vi "GDF File Reader.vi"() -> ()   [LabVIEW 2016]
uses:
  GDFv1.x File Reader/_vlib/GDFv1.x.lvclass
  GDFv1.x File Reader/_vlib/GDFv1.x.lvclass/GDFv1.x.ctl
  GDF File Reader.lvlib
panel:
  out "Application state info":string caption="Состояние обработки"
  in  "Stop Button":bool
  in  "Tab Control":enum32{"График ЭЭГ", "Таблица событий"}(tab)
  in  "Previous Dataset":bool
  in  "Next Dataset":bool
  out "EEG Graph":waveform(dbl)[](graph) caption="График ЭЭГ"
  out "Selected path":path caption="Путь к файлу"
  out "Sample Rate":dbl caption="Частота" format="%#_3f"
  out "Number of channels":i64 caption="Число каналов"
  out "Patient identificator":string="                                      " caption="Испытуемый"
  in  "Number of Trials in File":i32 caption="Число проб в XML файле"
  in  "Event Duration (in seconds)":dbl=1.0 caption="Продолжительность, с"
  out "Number of Events":i32 caption="Число проб выбранного типа"
  in  "Select Event Type":string(combo) caption="Выберите тип событий"
  in  "Save Events":bool caption="Сохранить пробы в XML"
  in  "Multicolumn Listbox":i32[](listbox) caption="Таблица событий"
  # "This VI is a part of BCI Design library, http://www.ru-bci.org \nCopyright © 2020, Sotnikov Peter, All rights reserved. License: GNU GPLv3"
  # "Hz"
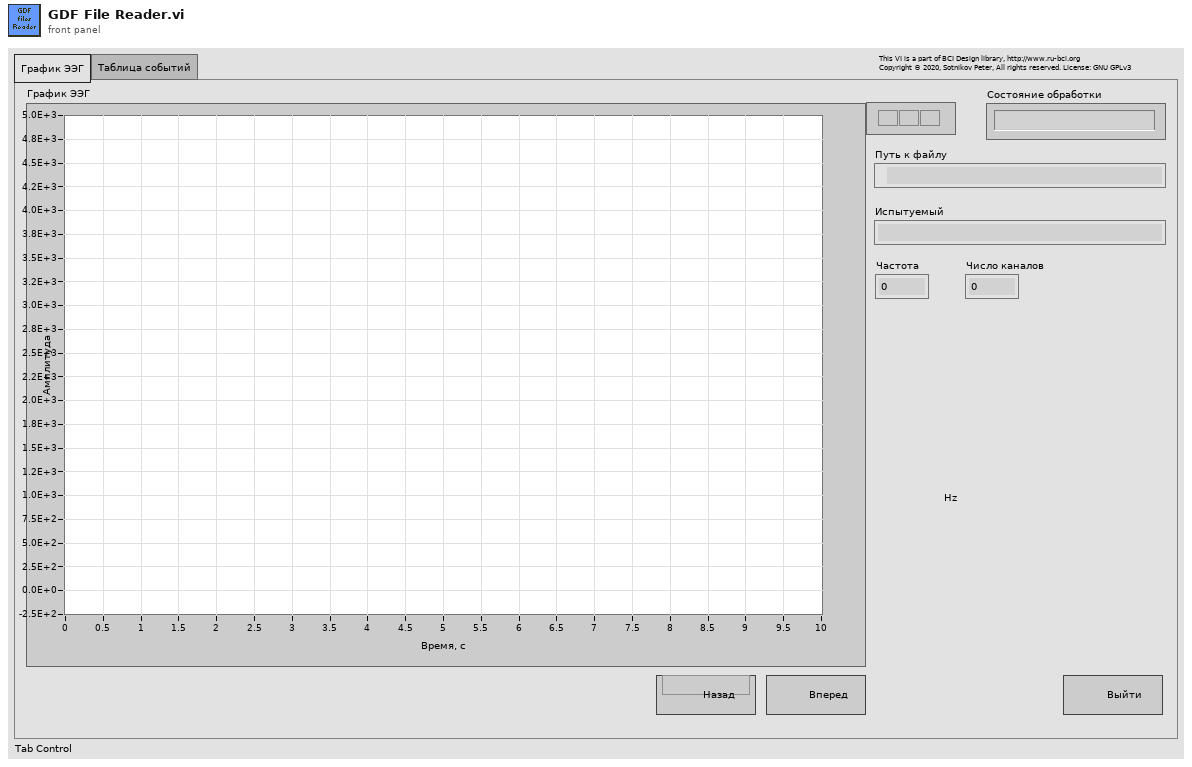
[diagram p1: front panel]
types:
  T1 = typedef "GDF File Reader.lvlib/GdfHeader1.ctl" = cluster{"Version identificator":string, "Patient identificator":string, "Recording identificator":string, "StartDateTime":timestamp, "Header record length":i64, "Equipment Provider":u64, "Laboratory":u64, "Technician":u64, "Number of data records":i64, "Duration of a data record":cluster{"Numerator":u32, "Denominator":u32}, "Number of signals":u32}
  T2 = typedef "GDF File Reader.lvlib/GdfHeader2.ctl" = cluster{"Channel labels":string[], "Transduser types":string[], "Physical dimensions":string[], "Physical lows":dbl[], "Physical highs":dbl[], "Digital lows":dbl[], "Digital highs":dbl[], "Channels Pre-filtering":string[], "Number of samples":u32[], "Channel types":u32[], "Addons":string[]}
  T3 = typedef "GDF File Reader.lvlib/EventDataType.ctl" = cluster{"Position (in samples)":u32, "EventType":string, "Channel":u16, "Duration (in samples)":u32}
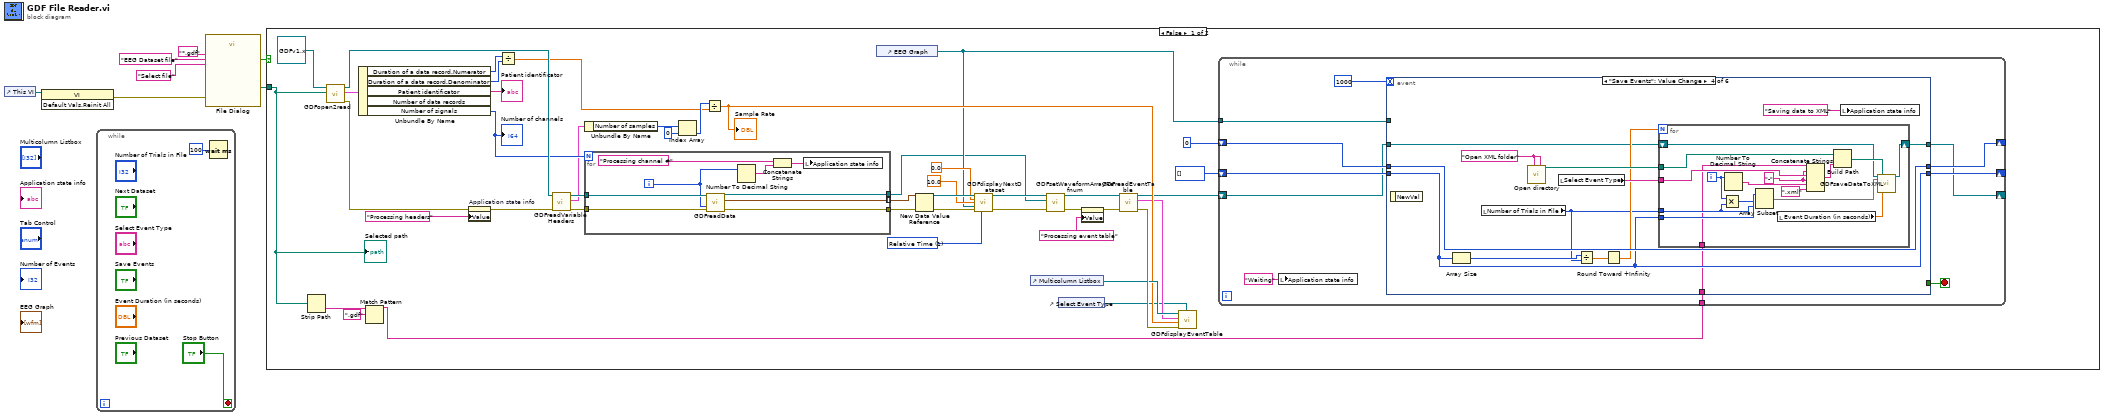
[diagram p0: block diagram]
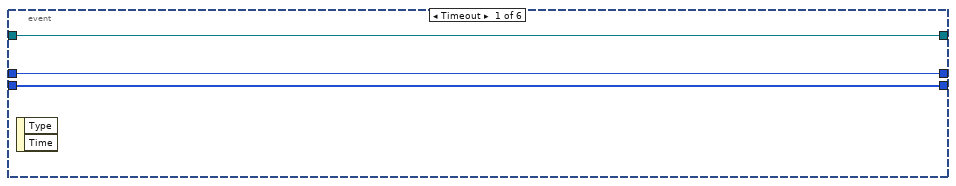
[diagram p2: hidden frame]
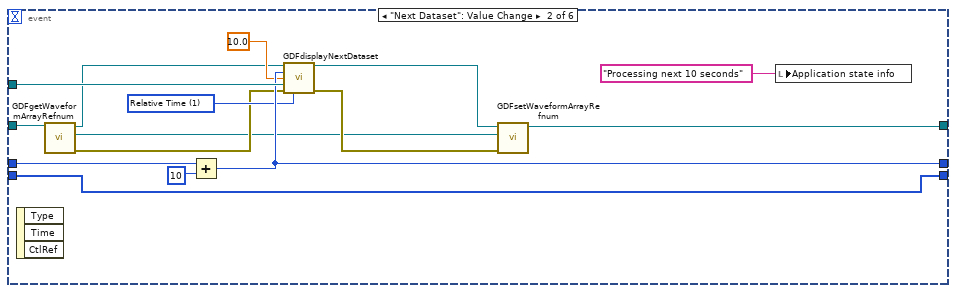
[diagram p3: hidden frame]
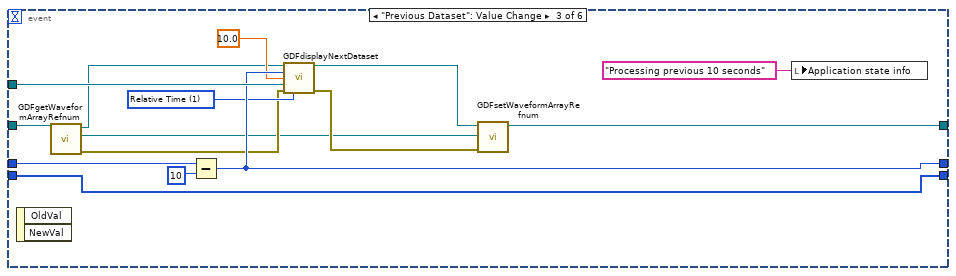
[diagram p4: hidden frame]
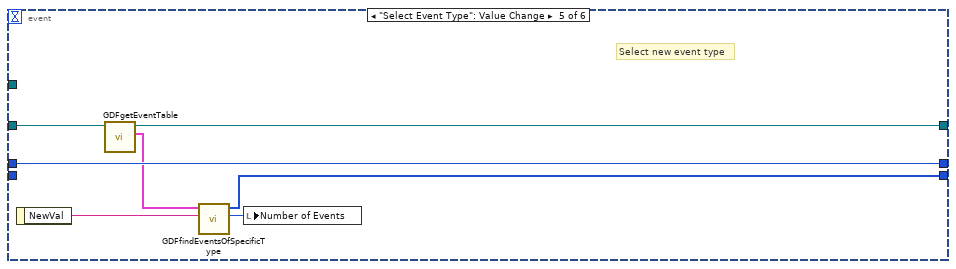
[diagram p5: hidden frame]
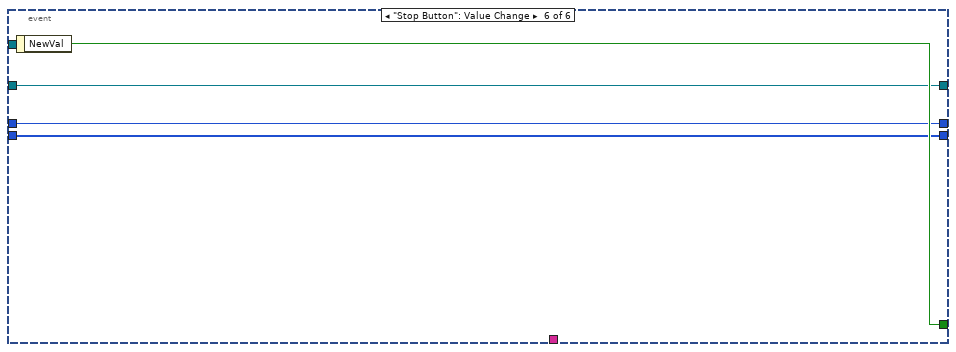
[diagram p6: hidden frame]
diagram:
  n1 = control-ref of="This VI"() -> (w2:refnum<vi>)
  n2 = invoke class="VI" method="Default Vals.Reinit All"(reference=w2) -> (error out=w1:errorcluster)  [unwired: 2 in, 2 out]
  n3 = while {
    stop <- "Stop Button" stop-if-true
    n4 = Wait (ms)(milliseconds to wait=u32 100) -> ()  [unwired: 1 out]
  }
  n5 = call "File Dialog"("button label"="Select file", "error in"=w1, "pattern (all files)"="*.gdf", "pattern label"="EEG Dataset file") -> ("selected path"=w4:path, "cancelled"=w5:bool)  [unwired: 8 in, 2 out]
  n6 = case shown="False" w5 {
    tunnel: w4 -> [w13 _]
    frame False {
      w24 = u16 1 items=["Samples", "Relative Time"] ("start/duration format")
      n7 = Strip Path(path=w13) -> (name=w12:string)  [unwired: 1 out]
      n8 = call "GDFopen2read.vi"("File path in"=w13, "GDFv1.x.lvclass in"=refnum<class "GDFv1.x.lvclass"> refnum ("GDFv1.x.lvclass")) -> ("error out"=w50:errorcluster, "GDF_header1"=w32:T1, "GDFv1.x.lvclass out"=w53:refnum<class "GDFv1.x.lvclass">)  [unwired: 7 in]
      n9 = Unbundle By Name(w32) -> ("Duration of a data record.Numerator"=w45:u32, "Duration of a data record.Denominator"=w44:u32, "Patient identificator"=→"Patient identificator":string, "Number of signals"=w36:u32)  [unwired: 1 out]
      "Number of channels" <- w36
      n10 = Match Pattern(string=w12, regular expression=".gdf") -> (before substring=w10:string)  [unwired: 1 in, 3 out]
      n11 = property on="Application state info" class="Str"(error in=w50, "Value"="Processing headers" ("Application state info")) -> (error out=w49:errorcluster)  [unwired: 1 in, 1 out]
      n12 = Divide(x=w45, y=w44) -> (x/y=w42:dbl)
      n13 = call "GDFreadVariableHeaders.vi"("error in"=w49, "GDFv1.x.lvclass in"=w53) -> ("error out"=w52:errorcluster, "GDFHeader2 out"=w31:T2, "GDFv1.x.lvclass out"=w51:refnum<class "GDFv1.x.lvclass">)  [unwired: 7 in]
      n14 = Unbundle By Name(w31) -> ("Number of samples"=w47:u32[])
      n15 = for {
        N: w36 -> [_]
        tunnel: w52 -> [w146]
        tunnel: w51 -> [w145]
        tunnel: [w144] -> w17
        tunnel: [w139] -> w30
        tunnel: [w138] -> w29 mode=indexing
        i -> [w141]
        n16 = call "GDFreadData.vi"("GDFv1.x.lvclass in"=w145, "Channel Number"=w141, "error in"=w146) -> ("GDFv1.x.lvclass out"=w144:refnum<class "GDFv1.x.lvclass">, "waveform out"=w138:waveform(dbl), "error out"=w139:errorcluster)  [unwired: 10 in]
        n17 = Number To Decimal String(number=w141) -> (decimal integer string=w140:string)  [unwired: 1 in]
        n18 = Concatenate Strings("Processing channel #" ("string"), w140) -> (w143:string)
        n19 = local write "Application state info"(w143) -> ()
      }
      n20 = Index Array(array=w47, index=0) -> (element=w43:u32)
      n21 = Divide(x=w43, y=w42) -> (x/y=w37:dbl)
      "Sample Rate" <- w37
      n22 = control-ref of="EEG Graph"() -> (w23:refnum<vi>)
      n23 = New Data Value Reference(data value=w29, error in=w30) -> (data value reference=w27:refnum<data-value>, error out=w28:errorcluster)
      n24 = call "GDFdisplayNextDataset.vi"("data value reference in"=w27, "Start"=0.0, "Duration"=10.0, "Waveform Graph Refnum in"=w23, "error in (no error)"=w28, "start/duration format"=w24) -> ("data value reference out"=w18:refnum<data-value>, "error out"=w20:errorcluster)  [unwired: 8 in]
      n25 = control-ref of="Multicolumn Listbox"() -> (w38:refnum<vi>)
      n26 = call "GDFsetWaveformArrayRefnum.vi"("error in (no error)"=w20, "GDFv1.x in"=w17, "Waveform Array Refnum in"=w18) -> ("error out"=w19:errorcluster, "GDFv1.x out"=w16:refnum<class "GDFv1.x.lvclass">)  [unwired: 7 in]
      n27 = control-ref of="Select Event Type"() -> (w22:refnum<vi>)
      n28 = property on="Application state info" class="Str"(error in=w19, "Value"="Processing event table") -> (error out=w34:errorcluster)  [unwired: 1 in, 1 out]
      n29 = call "GDFreadEventTable.vi"("error in"=w34, "GDFv1.x.lvclass in"=w16) -> ("error out"=w39:errorcluster, "Array of Events"=w33:T3[], "GDFv1.x.lvclass out"=w15:refnum<class "GDFv1.x.lvclass">)  [unwired: 6 in, 1 out]
      n30 = call "GDFdisplayEventTable.vi"("Select Event Type"=w22, "error in (no error)"=w39, "Samplerate"=w37, "Array of Events in"=w33, "Multicolumn Listbox in"=w38) -> ()  [unwired: 6 in, 1 out]
      n31 = while {
        shift-right: [w62] -> _
        shift-left: 0 -> [w61]
        tunnel: w23 -> [w59]
        shift-right: [w57] -> _
        shift-left: i32[] [] -> [w58]
        shift-right: [w55] -> _
        shift-left: w15 -> [w56]
        tunnel: w10 -> [w54]
        stop <- w63 stop-if-true
        n32 = local write "Application state info"("Waiting" ("Application state info")) -> ()
        n33 = event shown="[3] \"Save Events\": Value Change" {
          selector: _ -> [_ _ _ _ _ _]
          dyn-events: _ -> [_ _ _ _ _ _]
          timeout: 1000 -> [_ _ _ _ _ _]
          tunnel: [_ _ _ _ _ w137] -> w63
          tunnel: [w67 w78 w93 w110 w133 w136] -> w62
          tunnel: w61 -> [w67 w81 w95 w110 w133 w136]
          tunnel: w59 -> [_ w79 w96 _ _ _]
          tunnel: w58 -> [w66 w75 w90 w103 _ w135]
          tunnel: [w66 w75 w90 w103 w130 w135] -> w57
          tunnel: w56 -> [w65 w74 w89 w100 w129 w134]
          tunnel: [w65 w70 w85 w99 w127 w134] -> w55
          tunnel: w54 -> [_ _ _ w98 _ _]
          event Timeout {
            n34 = event-data() -> ()  [unwired: 1 in, 2 out]
          }
          event "Next Dataset": Value Change {
            w77 = u16 1 items=["Samples", "Relative Time"] ("start/duration format")
            n35 = event-data() -> ()  [unwired: 1 in, 3 out]
            n36 = call "GDFgetWaveformArrayRefnum.vi"("GDFv1.x in"=w74) -> ("error out"=w72:errorcluster, "GDFv1.x out"=w68:refnum<class "GDFv1.x.lvclass">, "Waveform array reference"=w69:refnum<data-value>)  [unwired: 8 in]
            n37 = Add(x=w81, y=10) -> (x+y=w78:i32)
            n38 = call "GDFdisplayNextDataset.vi"("data value reference in"=w69, "Start"=w78, "Duration"=10.0, "Waveform Graph Refnum in"=w79, "error in (no error)"=w72, "start/duration format"=w77) -> ("data value reference out"=w73:refnum<data-value>, "error out"=w71:errorcluster)  [unwired: 8 in]
            n39 = call "GDFsetWaveformArrayRefnum.vi"("error in (no error)"=w71, "GDFv1.x in"=w68, "Waveform Array Refnum in"=w73) -> ("GDFv1.x out"=w70:refnum<class "GDFv1.x.lvclass">)  [unwired: 7 in, 1 out]
            n40 = local write "Application state info"("Processing next 10 seconds" ("Application state info")) -> ()
          }
          event "Previous Dataset": Value Change {
            w91 = u16 1 items=["Samples", "Relative Time"] ("start/duration format")
            n41 = event-data() -> ()  [unwired: 1 in, 2 out]
            n42 = call "GDFgetWaveformArrayRefnum.vi"("GDFv1.x in"=w89) -> ("error out"=w88:errorcluster, "GDFv1.x out"=w83:refnum<class "GDFv1.x.lvclass">, "Waveform array reference"=w84:refnum<data-value>)  [unwired: 8 in]
            n43 = Subtract(x=w95, y=10) -> (x-y=w93:i32)
            n44 = call "GDFdisplayNextDataset.vi"("data value reference in"=w84, "Start"=w93, "Duration"=10.0, "Waveform Graph Refnum in"=w96, "error in (no error)"=w88, "start/duration format"=w91) -> ("data value reference out"=w86:refnum<data-value>, "error out"=w87:errorcluster)  [unwired: 8 in]
            n45 = call "GDFsetWaveformArrayRefnum.vi"("error in (no error)"=w87, "GDFv1.x in"=w83, "Waveform Array Refnum in"=w86) -> ("GDFv1.x out"=w85:refnum<class "GDFv1.x.lvclass">)  [unwired: 7 in, 1 out]
            n46 = local write "Application state info"("Processing previous 10 seconds" ("Application state info")) -> ()
          }
          event "Save Events": Value Change {
            w101 = "Open XML folder" ("default name")
            n47 = event-data() -> ()  [unwired: 1 in, 1 out]
            n48 = Array Size(array=w103) -> (size(s)=w106:i32)
            n49 = local read "Number of Trials in File"() -> (w102:i32)
            n50 = call "Open directory"("prompt"=w101, "button label"=w101) -> ("selected path"=w107:path)  [unwired: 10 in, 3 out]
            n51 = local read "Select Event Type"() -> (w108:string)
            n52 = Divide(x=w106, y=w102) -> (x/y=w105:dbl)
            n53 = Round Toward +Infinity(x=w105) -> (ceil(x): smallest int >= x=w104:dbl)
            n54 = for {
              N: w104 -> [_]
              tunnel: w108 -> [w126]
              tunnel: w107 -> [w123]
              tunnel: w103 -> [w120]
              tunnel: w102 -> [w117]
              shift-right: [w113] -> w99
              shift-left: w100 -> [w114]
              tunnel: w98 -> [w111]
              i -> [w118]
              w112 = "-" ("string")
              n55 = Multiply(x=w118, y=w117) -> (x*y=w119:i32)
              n56 = Number To Decimal String(number=w118) -> (decimal integer string=w125:string)  [unwired: 1 in]
              n57 = Array Subset(array=w120, index=w119, length=w117) -> (w116:i32[])
              n58 = local read "Event Duration (in seconds)"() -> (w115:dbl)
              n59 = Concatenate Strings(w111, w112, w126, w112, w125, ".xml" ("string")) -> (w122:string)
              n60 = Build Path(base path=w123, name or relative path=w122) -> (appended path=w121:path)
              n61 = call "GDFsaveDataToXML.vi"("GDFv1.x.lvclass"=w114, "Array of indexes"=w116, "XML file path"=w121, "Duration"=w115) -> ("output cluster"=w113:refnum<class "GDFv1.x.lvclass">)  [unwired: 14 in, 1 out]
            }
            n62 = local write "Application state info"("Saving data to XML" ("Application state info")) -> ()
          }
          event "Select Event Type": Value Change {
            # "Select new event type"
            n63 = event-data() -> ("NewVal"=w132:string)  [unwired: 1 in]
            n64 = call "GDFgetEventTable.vi"("GDFv1.x in"=w129) -> ("Event Table"=w128:T3[], "GDFv1.x out"=w127:refnum<class "GDFv1.x.lvclass">)  [unwired: 8 in, 1 out]
            n65 = call "GDFfindEventsOfSpecificType.vi"("Selected Event Type"=w132, "Array of Events in"=w128) -> ("Number Of Events"=w131:i32, "Array of Event Indexes"=w130:i32[])  [unwired: 8 in]
            n66 = local write "Number of Events"(w131) -> ()
          }
          event "Stop Button": Value Change {
            n67 = event-data() -> ("NewVal"=w137:bool)  [unwired: 1 in]
          }
        }
      }
      "Selected path" <- w13
    }
    frame True {
    }
  }
